vi "Find Next XML Element.vi"(8 "error in (no error)":errorcluster, 11 "XML Fine In":refnum<file>) -> (0 "error out":errorcluster, 2 "Comment":string, 3 "XML Fine Out":refnum<file>)   [LabVIEW 2013, in "XML Parser.lvclass"]
uses:
  XML Parser.lvclass
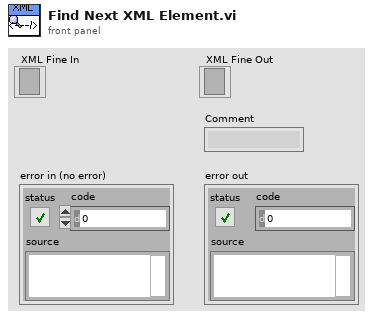
[diagram p1: front panel]
types:
  T1 = typedef "XML Parser.lvclass/XML element Types.ctl" = enum16{"Element", "Comment", "Empty Line"}
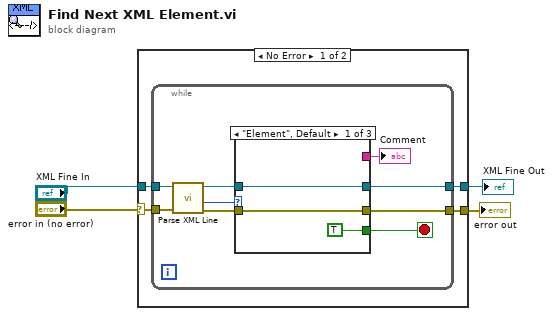
[diagram p0: block diagram]
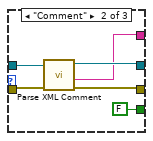
[diagram p2: hidden frame]
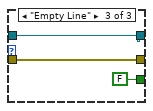
[diagram p3: hidden frame]
diagram:
  n1 = case shown="No Error" "error in (no error)" {
    selector: "error in (no error)" -> [w5 w31]
    tunnel: [w8 w31] -> w4
    tunnel: [w7 w30] -> w3
    tunnel: "XML Fine In" -> [w6 w30]
    frame No Error {
      n2 = while {
        tunnel: w5 -> [w17]
        tunnel: w6 -> [w16]
        tunnel: [w12] -> w7
        tunnel: [w11] -> w8
        stop <- w14 stop-if-true
        n3 = call "Parse XML Line.vi"("error in (no error)"=w17, "XML Refnum in"=w16) -> ("error out"=w10:errorcluster, "Line Type"=w15:T1, "XML Refnum out"=w13:refnum<file>)  [unwired: 7 in]
        n4 = case shown="\"Element\", Default" w15 {
          tunnel: [TRUE FALSE FALSE] -> w14
          tunnel: [w19 w23 w28] -> w12
          tunnel: w13 -> [w19 w26 w28]
          tunnel: [w18 w24 w29] -> w11
          tunnel: w10 -> [w18 w25 w29]
          tunnel: [_ w21 _] -> w9
          frame "Element", Default {
          }
          frame "Comment" {
            n5 = call "Parse XML Comment.vi"("error in (no error)"=w25, "XML Refnum in"=w26) -> ("error out"=w24:errorcluster, "Comment"=w21:string, "XML Refnum out"=w23:refnum<file>)  [unwired: 6 in, 1 out]
          }
          frame "Empty Line" {
          }
        }
        "Comment" <- w9
      }
    }
    frame Error {
    }
  }
  "error out" <- w4
  "XML Fine Out" <- w3
